vi "MKS CTLR - Config Serial Port.vi"(8 "Error In":errorcluster, 11 "MKS ViiSA resource name in":refnum<visa-resource-name>) -> (0 "Error Out":errorcluster, 3 "VISA resource name out":refnum<visa-resource-name>)   [LabVIEW 2013]
uses:
  MKS CTLR - Serial parameters.ctl
  <vilib>/Instr/_visa.llb/VISA Flush IO Buffer Mask.ctl
  <vilib>/Instr/_visa.llb/VISA Configure Serial Port (Instr).vi
panel:
  in  "MKS Controller Parameters":T1={"VISA resource name"="", "Baud rate"=enum."9600", "Parity"=enum."None", "Stop Bits"=enum."1", "Flow Control"=enum."None", "Data bits "=8, "Timeout (Sec)"=10, "termination char"=10, "Enable Termination"=TRUE} {"termination char" format="%.0x"; "Data bits" min=7 max=8 step=1}
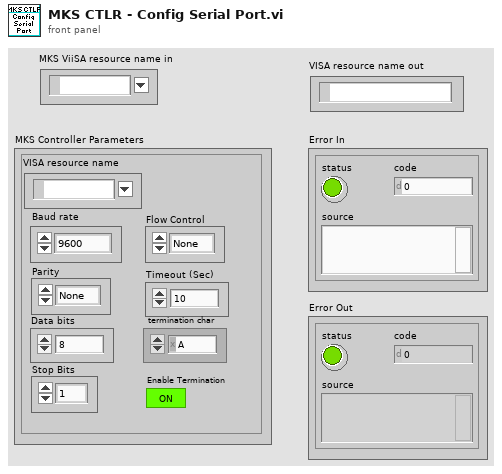
[diagram p1: front panel]
types:
  T1 = typedef "MKS CTLR - Serial parameters.ctl" = cluster{"VISA resource name":refnum<visa-resource-name>, "Baud rate":enum16{"300", "1200", "2400", "4800", "9600", "19200", "38400", "57600", "115200"}, "Parity":enum16{"None", "Odd", "Even", "Mark", "Space"}, "Stop Bits":enum16{"1", "1.5", "2"}, "Flow Control":enum16{"None", "X-OFF", "RTS / CTS"}, "Data bits ":u16, "Timeout (Sec)":u32, "termination char":u8, "Enable Termination":bool}
  T2 = typedef "VISA Flush IO Buffer Mask.ctl" = u16
  T3 = enum16{"300", "1200", "2400", "4800", "9600", "19200", "38400", "57600", "115200"}
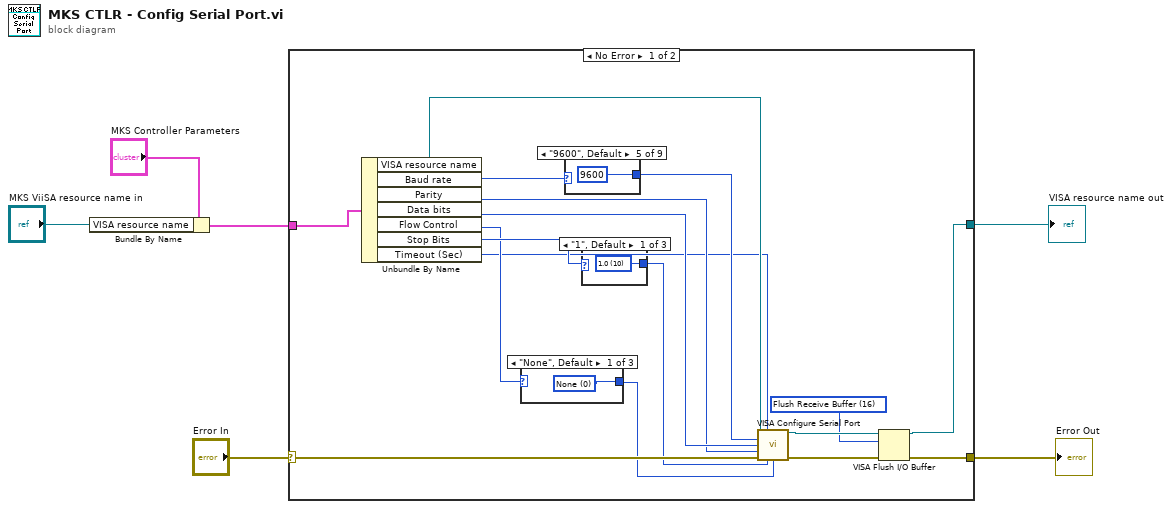
[diagram p0: block diagram]
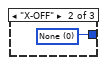
[diagram p2: hidden frame]
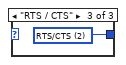
[diagram p3: hidden frame]
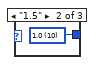
[diagram p4: hidden frame]
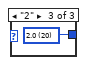
[diagram p5: hidden frame]
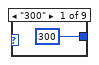
[diagram p6: hidden frame]
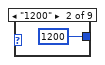
[diagram p7: hidden frame]
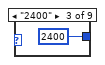
[diagram p8: hidden frame]
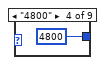
[diagram p9: hidden frame]
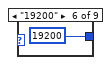
[diagram p10: hidden frame]
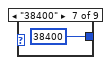
[diagram p11: hidden frame]
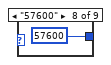
[diagram p12: hidden frame]
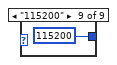
[diagram p13: hidden frame]
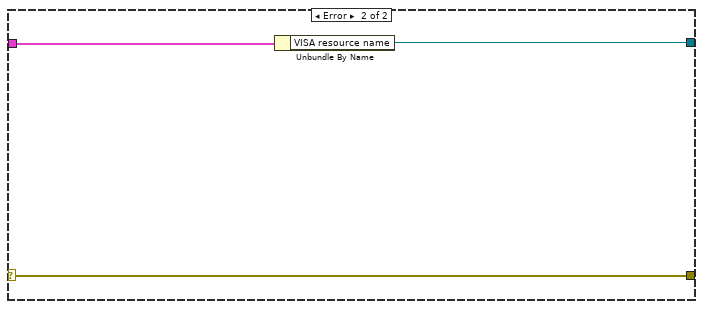
[diagram p14: hidden frame]
diagram:
  n1 = Bundle By Name(cluster="MKS Controller Parameters", "VISA resource name"="MKS ViiSA resource name in") -> (w1:T1)
  n2 = case shown="No Error" "Error In" {
    selector: "Error In" -> [w17 w39]
    tunnel: [w8 w39] -> w6
    tunnel: w1 -> [w22 w41]
    tunnel: [w9 w40] -> w4
    frame No Error {
      w7 = T2 16 items=["Flush Receive Buffer"=16, "Write Transmit Buffer to Device"=32, "Flush Receive Buffer (No I/O)"=64, "Flush Transmit Buffer"=128] ("Mask")
      n3 = Unbundle By Name(w22) -> ("VISA resource name"=w20:refnum<visa-resource-name>, "Baud rate"=w21:T3, "Parity"=w18:enum16{"None", "Odd", "Even", "Mark", "Space"}, "Data bits"=w19:u16, "Flow Control"=w14:enum16{"None", "X-OFF", "RTS / CTS"}, "Stop Bits"=w23:enum16{"1", "1.5", "2"}, "Timeout (Sec)"=w12:u32)
      n4 = case shown="\"None\", Default" w14 {
        tunnel: [w24 w25 w26] -> w13
        frame "None", Default {
          w24 = u16 0 items=["None", "XON/XOFF", "RTS/CTS", "XON/XOFF & RTS/CTS", "DTR/DSR", "XON/XOFF & DTR/DSR"] ("flow control (0:none)")
        }
        frame "X-OFF" {
          w25 = u16 0 items=["None", "XON/XOFF", "RTS/CTS", "XON/XOFF & RTS/CTS", "DTR/DSR", "XON/XOFF & DTR/DSR"] ("flow control (0:none)")
        }
        frame "RTS / CTS" {
          w26 = u16 2 items=["None", "XON/XOFF", "RTS/CTS", "XON/XOFF & RTS/CTS", "DTR/DSR", "XON/XOFF & DTR/DSR"] ("flow control (0:none)")
        }
      }
      n5 = case shown="\"9600\", Default" w21 {
        tunnel: [300 1200 2400 u32 4800 u32 9600 u32 19200 u32 38400 u32 57600 u32 115200] -> w16
        frame "300" {
        }
        frame "1200" {
        }
        frame "2400" {
        }
        frame "4800" {
        }
        frame "9600", Default {
        }
        frame "19200" {
        }
        frame "38400" {
        }
        frame "57600" {
        }
        frame "115200" {
        }
      }
      n6 = case shown="\"1\", Default" w23 {
        tunnel: [w27 w28 w29] -> w15
        frame "1", Default {
          w27 = u16 10 items=["1.0"=10, "1.5"=15, "2.0"=20] ("stop bits (10: 1 bit)")
        }
        frame "1.5" {
          w28 = u16 10 items=["1.0"=10, "1.5"=15, "2.0"=20] ("stop bits (10: 1 bit)")
        }
        frame "2" {
          w29 = u16 20 items=["1.0"=10, "1.5"=15, "2.0"=20] ("stop bits (10: 1 bit)")
        }
      }
      n7 = call-poly "VISA Configure Serial Port"("VISA resource name"=w20, "timeout (10sec)"=w12, "baud rate (9600)"=w16, "data bits (8)"=w19, "parity (0:none)"=w18, "error in (no error)"=w17, "stop bits (10: 1 bit)"=w15, "flow control (0:none)"=w13) -> ("VISA resource name out"=w10:refnum<visa-resource-name>, "error out"=w11:errorcluster)  [unwired: 6 in]
      n8 = VISA Flush I/O Buffer(VISA resource name=w10, mask (16)=w7, error in (no error)=w11) -> (VISA resource name out=w9:refnum<visa-resource-name>, error out=w8:errorcluster)
    }
    frame Error {
      n9 = Unbundle By Name(w41) -> ("VISA resource name"=w40:refnum<visa-resource-name>)
    }
  }
  "Error Out" <- w6
  "VISA resource name out" <- w4
